vi "KlingerV2 ReadPosition.vi"(8 "error in":errorcluster, 9 "UnitDem":u8(ring)=2 caption="Unités" items=["Pas", "mm", "ps", "Degré (°)"], 10 "Axe":u8(ring) items=["W", "X", "Y", "Z"], 11 "VISA Rsrc":refnum<visa-resource-name>="SR530") -> (0 "error out":errorcluster, 1 "Cont Error":string caption="Message d'erreur", 2 "Statut":bool, 3 "Position":dbl format="%^#_9e", 4 "NLimit":bool caption="Limite -", 5 "Moving":bool caption="Déplacement\nen cours", 6 "PLimit":bool caption="Limite +")   [LabVIEW 2012]
doc: "Ce VI retourne la position de l'axe moteur spécifié dans l'unité indiquée. Il retourne aussi l'état des interrupteurs de fin de course sur cet axe et indique si un déplacement y est en cours."
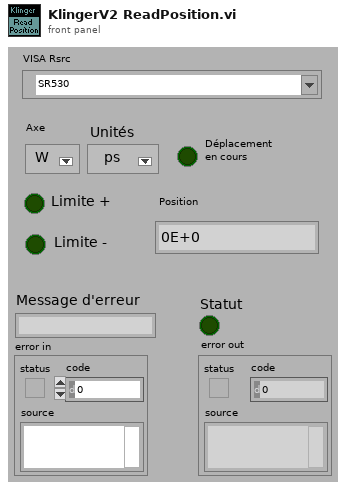
[diagram p1: front panel]
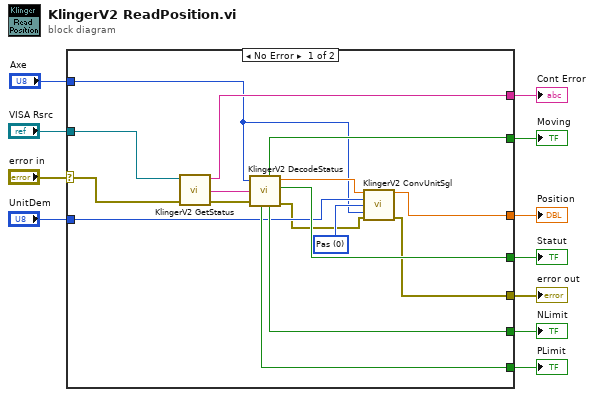
[diagram p0: block diagram]
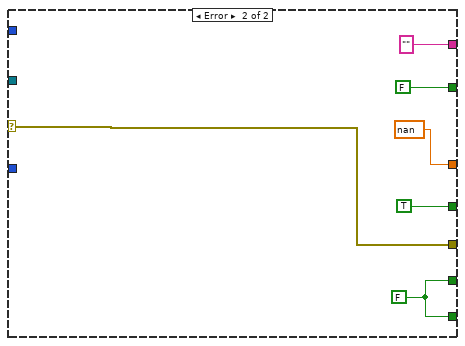
[diagram p2: hidden frame]
diagram:
  n1 = case shown="No Error" "error in" {
    selector: "error in" -> [w12 w32]
    tunnel: [w24 w28] -> w11
    tunnel: [w25 w28] -> w10
    tunnel: [w17 nan] -> w9
    tunnel: "Axe" -> [w16 _]
    tunnel: [w14 w32] -> w7
    tunnel: [w21 "" ("Message D'erreur")] -> w6
    tunnel: [w26 TRUE ("Statut")] -> w5
    tunnel: [w23 FALSE] -> w3
    tunnel: "UnitDem" -> [w19 _]
    tunnel: "VISA Rsrc" -> [w13 _]
    frame No Error {
      w20 = u8 0 items=["Pas", "mm", "ps"] ("UnitAct")
      n2 = call <userlib>:"KlingerV2 GetStatus.vi"("error in"=w12, "VISA Rsrc"=w13) -> ("error out"=w22:errorcluster, "Message Cont"=w27:string, "Message D'erreur"=w21:string)  [unwired: 2 in, 1 out]
      n3 = call <userlib>:"KlingerV2 DecodeStatus.vi"("Axe"=w16, "Message Cont"=w27, "error in"=w22) -> ("PLimit"=w24:bool, "Moving"=w23:bool, "Position"=w18:dbl, "Statut"=w26:bool, "NLimit"=w25:bool, "error out"=w15:errorcluster)  [unwired: 2 in]
      n4 = call <userlib>:"KlingerV2 ConvUnitSgl.vi"("ParamAct"=w18, "UnitDem"=w19, "UnitAct"=w20, "Axe"=w16, "error in"=w15) -> ("ParamDem"=w17:dbl, "error out"=w14:errorcluster)  [unwired: 9 in]
    }
    frame Error {
      w28 = FALSE
    }
  }
  "Moving" <- w3
  "PLimit" <- w11
  "NLimit" <- w10
  "Position" <- w9
  "Cont Error" <- w6
  "error out" <- w7
  "Statut" <- w5
